vi "GV line gate.vi"() -> ()   [LabVIEW 2017]
panel:
  out "Line gate":bool
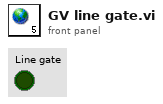
[diagram p1: front panel]
diagram:
